vi "Insert Into SubPanel.vi"(8 "error in (no error)":errorcluster, 10 "SubPanel Ref":refnum<vi>, 11 "Actor wUI in":refnum<class "Actor wUI.lvclass">) -> (0 "error out":errorcluster, 3 "Actor wUI out":refnum<class "Actor wUI.lvclass">)   [LabVIEW 2017, in "Framework.lvlib" / "Actor wUI.lvclass"]
uses:
  Actor wUI.lvclass
  Actor wUI.lvclass/Actor wUI.ctl
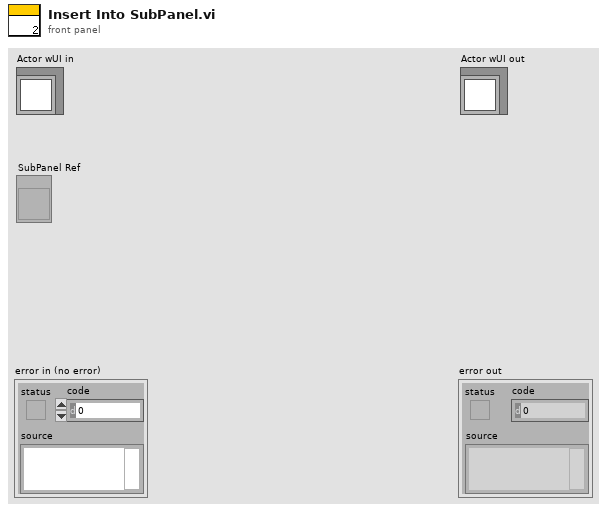
[diagram p1: front panel]
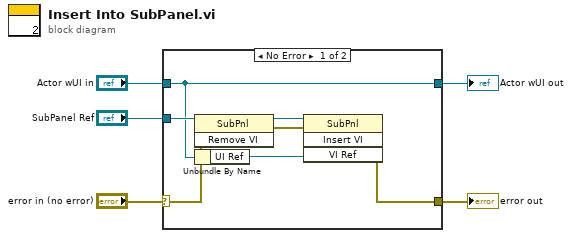
[diagram p0: block diagram]
diagram:
  n1 = case shown="No Error" "error in (no error)" {
    selector: "error in (no error)" -> [w7 w14]
    tunnel: [w6 w14] -> w4
    tunnel: [w9 w13] -> w2
    tunnel: "Actor wUI in" -> [w9 w13]
    tunnel: "SubPanel Ref" -> [w10 _]
    frame No Error {
      n2 = invoke class="SubPnl" method="Remove VI"(reference=w10, error in=w7) -> (reference out=w12:refnum<vi>, error out=w11:errorcluster)  [unwired: 1 in, 1 out]
      n3 = Unbundle By Name(w9) -> ("UI Ref"=w8:refnum<vi>)
      n4 = invoke class="SubPnl" method="Insert VI"(reference=w12, error in=w11, "VI Ref"=w8) -> (error out=w6:errorcluster)  [unwired: 1 in, 3 out]
    }
    frame Error {
    }
  }
  "error out" <- w4
  "Actor wUI out" <- w2
